vi "XML-compresion con etiquetas.vi"() -> ()   [LabVIEW 2010]
panel:
  out "temp 2":string="<?xml version=\"1.0\" encoding=\"UTF-8\"?><methodCall><methodName>jil.syncvi</methodName><params><param><value><array><value><struct><member><name>name</name><value><string>intin</string></value></member><member><name>action</name><value><string>set</string></value></member><member><name>value</name><value><int>0</int></value></member></struct></value><value><struct><member><name>name</name><value><string>doublein</string></value></member><member><name>action</name><value><string>set</string></value></member><member><name>value</name><value><double>0,000000</double></value></member></struct></value><value><struct><member><name>name</name><value><string>booleanin</string></value></member><member><name>action</name><value><string>set</string></value></member><member><name>value</name><value><boolean>1</boolean></value></member></struct></value><value><struct><member><name>name</name><value><string>stringin</string></value></member><member><name>action</name><value><string>set</string></value></member><member><name>value</name><value><string></string></value></member></struct></value><value><struct><member><name>name</name><value><string>intout</string></value></member><member><name>action</name><value><string>get</string></value></member><member><name>value</name><value><int>0</int></value></member></struct></value><value><struct><member><name>name</name><value><string>doubleout</string></value></member><member><name>action</name><value><string>get</string></value></member><member><name>value</name><value><double>0</double></value></member></struct></value><value><struct><member><name>name</name><value><string>booleanout</string></value></member><member><name>action</name><value><string>get</string></value></member><member><name>value</name><value><boolean>0</boolean></value></member></struct></value><value><struct><member><name>name</name><value><string>stringout</string></value></member><member><name>action</name><value><string>get</string></value></member><member><name>value</name><value><string>a</string></value></member></struct></value></array></value></param></params></methodCall>"
  out "temp":string="<1>intin<2>set<3><8>0</8><4>doublein<2>set<3><6>0,000000</6><4>booleanin<2>set<3><5>1</5><4>stringin<2>set<3><7></7><4>intout<2>get<3><8>0</8><4>doubleout<2>get<3><6>0</6><4>booleanout<2>get<3><5>0</5><4>stringout<2>get<3><7>a</7></1>"
  in  "comprimido":string[](array[string])=["<1>", "</1>", "<2>", "<3>", "<4>", "<5>", "</5>", "<6>", "</6>", "<7>", "</7>", "<8>", "</8>"]
  in  "Expandido":string[](array[string])=["<?xml version=\"1.0\" encoding=\"UTF-8\"?><methodCall><methodName>jil.syncvi</methodName><params><param><value><array><value><struct><member><name>name</name><value><string>", "</value></member></struct></value></array></value></param></params></methodCall>", "</string></value></member><member><name>action</name><value><string>", "</string></value></member><member><name>value</name><value>", "</value></member></struct></value><value><struct><member><name>name</name><value><string>", "<boolean>", "</boolean>", "<double>", "</double>", "<string>", "</string>", "<int>", "</int>"]
  out "antes 2":string="<?xml version=\"1.0\" encoding=\"UTF-8\"?>\n<methodCall>\n<methodName>jil.syncvi</methodName>\n<params>\n<param>\n<value>\n<array>\n<value>\n<struct>\n<member>\n<name>name</name>\n<value>\n<string>intin</string>\n</value>\n</member>\n<member>\n<name>action</name>\n<value>\n<string>set</string>\n</value>\n</member>\n<member>\n<name>value</name>\n<value>\n<int>0</int>\n</value>\n</member>\n</struct>\n</value>\n<value>\n<struct>\n<member>\n<name>name</name>\n<value>\n<string>doublein</string>\n</value>\n</member>\n<member>\n<name>action</name>\n<value>\n<string>set</string>\n</value>\n</member>\n<member>\n<name>value</name>\n<value>\n<double>0,000000</double>\n</value>\n</member>\n</struct>\n</value>\n<value>\n<struct>\n<member>\n<name>name</name>\n<value>\n<string>booleanin</string>\n</value>\n</member>\n<member>\n<name>action</name>\n<value>\n<string>set</string>\n</value>\n</member>\n<member>\n<name>value</name>\n<value>\n<boolean>1</boolean>\n</value>\n</member>\n</struct>\n</value>\n<value>\n<struct>\n<member>\n<name>name</name>\n<value>\n<string>stringin</string>\n</value>\n</member>\n<member>\n<name>action</name>\n<value>\n<string>set</string>\n</value>\n</member>\n<member>\n<name>value</name>\n<value>\n<string></string>\n</value>\n</member>\n</struct>\n</value>\n<value>\n<struct>\n<member>\n<name>name</name>\n<value>\n<string>intout</string>\n</value>\n</member>\n<member>\n<name>action</name>\n<value>\n<string>get</string>\n</value>\n</member>\n<member>\n<name>value</name>\n<value>\n<int>0</int>\n</value>\n</member>\n</struct>\n</value>\n<value>\n<struct>\n<member>\n<name>name</name>\n<value>\n<string>doubleout</string>\n</value>\n</member>\n<member>\n<name>action</name>\n<value>\n<string>get</string>\n</value>\n</member>\n<member>\n<name>value</name>\n<value>\n<double>0</double>\n</value>\n</member>\n</struct>\n</value>\n<value>\n<struct>\n<member>\n<name>name</name>\n<value>\n<string>booleanout</string>\n</value>\n</member>\n<member>\n<name>action</name>\n<value>\n<string>get</string>\n</value>\n</member>\n<member>\n<name>value</name>\n<value>\n<boolean>0</boolean>\n</value>\n</member>\n</struct>\n</value>\n<value>\n<struct>\n<member>\n<name>name</name>\n<value>\n<string>stringout</string>\n</value>\n</member>\n<member>\n<name>action</name>\n<value>\n<string>get</string>\n</value>\n</member>\n<member>\n<name>value</name>\n<value>\n<string>a</string>\n</value>\n</member>\n</struct>\n</value>\n</array>\n</value>\n</param>\n</params>\n</methodCall>"
  out "despues 2":string
  out "despues":string
  out "Mensaje LEGIBLE DESC":string="<?xml version=\"1.0\" encoding=\"UTF-8\"?>\n<methodCall>\n<methodName>jil.syncvi</methodName>\n<params>\n<param>\n<value>\n<array>\n<value>\n<struct>\n<member>\n<name>name</name>\n<value>\n<string>intin</string>\n</value>\n</member>\n<member>\n<name>action</name>\n<value>\n<string>set</string>\n</value>\n</member>\n<member>\n<name>value</name>\n<value>\n<int>0</int>\n</value>\n</member>\n</struct>\n</value>\n<value>\n<struct>\n<member>\n<name>name</name>\n<value>\n<string>doublein</string>\n</value>\n</member>\n<member>\n<name>action</name>\n<value>\n<string>set</string>\n</value>\n</member>\n<member>\n<name>value</name>\n<value>\n<double>0,000000</double>\n</value>\n</member>\n</struct>\n</value>\n<value>\n<struct>\n<member>\n<name>name</name>\n<value>\n<string>booleanin</string>\n</value>\n</member>\n<member>\n<name>action</name>\n<value>\n<string>set</string>\n</value>\n</member>\n<member>\n<name>value</name>\n<value>\n<boolean>1</boolean>\n</value>\n</member>\n</struct>\n</value>\n<value>\n<struct>\n<member>\n<name>name</name>\n<value>\n<string>stringin</string>\n</value>\n</member>\n<member>\n<name>action</name>\n<value>\n<string>set</string>\n</value>\n</member>\n<member>\n<name>value</name>\n<value>\n<string></string>\n</value>\n</member>\n</struct>\n</value>\n<value>\n<struct>\n<member>\n<name>name</name>\n<value>\n<string>intout</string>\n</value>\n</member>\n<member>\n<name>action</name>\n<value>\n<string>get</string>\n</value>\n</member>\n<member>\n<name>value</name>\n<value>\n<int>0</int>\n</value>\n</member>\n</struct>\n</value>\n<value>\n<struct>\n<member>\n<name>name</name>\n<value>\n<string>doubleout</string>\n</value>\n</member>\n<member>\n<name>action</name>\n<value>\n<string>get</string>\n</value>\n</member>\n<member>\n<name>value</name>\n<value>\n<double>0</double>\n</value>\n</member>\n</struct>\n</value>\n<value>\n<struct>\n<member>\n<name>name</name>\n<value>\n<string>booleanout</string>\n</value>\n</member>\n<member>\n<name>action</name>\n<value>\n<string>get</string>\n</value>\n</member>\n<member>\n<name>value</name>\n<value>\n<boolean>0</boolean>\n</value>\n</member>\n</struct>\n</value>\n<value>\n<struct>\n<member>\n<name>name</name>\n<value>\n<string>stringout</string>\n</value>\n</member>\n<member>\n<name>action</name>\n<value>\n<string>get</string>\n</value>\n</member>\n<member>\n<name>value</name>\n<value>\n<string>a</string>\n</value>\n</member>\n</struct>\n</value>\n</array>\n</value>\n</param>\n</params>\n</methodCall>"
  out "Tiempo que tarda\nen comprimir y descomorimir (ms)":dbl=1.068
  out "OK?":bool=TRUE
  out "MensajeDESC":string="<?xml version=\"1.0\" encoding=\"UTF-8\"?><methodCall><methodName>jil.syncvi</methodName><params><param><value><array><value><struct><member><name>name</name><value><string>intin</string></value></member><member><name>action</name><value><string>set</string></value></member><member><name>value</name><value><int>0</int></value></member></struct></value><value><struct><member><name>name</name><value><string>doublein</string></value></member><member><name>action</name><value><string>set</string></value></member><member><name>value</name><value><double>0,000000</double></value></member></struct></value><value><struct><member><name>name</name><value><string>booleanin</string></value></member><member><name>action</name><value><string>set</string></value></member><member><name>value</name><value><boolean>1</boolean></value></member></struct></value><value><struct><member><name>name</name><value><string>stringin</string></value></member><member><name>action</name><value><string>set</string></value></member><member><name>value</name><value><string></string></value></member></struct></value><value><struct><member><name>name</name><value><string>intout</string></value></member><member><name>action</name><value><string>get</string></value></member><member><name>value</name><value><int>0</int></value></member></struct></value><value><struct><member><name>name</name><value><string>doubleout</string></value></member><member><name>action</name><value><string>get</string></value></member><member><name>value</name><value><double>0</double></value></member></struct></value><value><struct><member><name>name</name><value><string>booleanout</string></value></member><member><name>action</name><value><string>get</string></value></member><member><name>value</name><value><boolean>0</boolean></value></member></struct></value><value><struct><member><name>name</name><value><string>stringout</string></value></member><member><name>action</name><value><string>get</string></value></member><member><name>value</name><value><string>a</string></value></member></struct></value></array></value></param></params></methodCall>"
  out "length 3":i32=234
  out "Mensaje3":string="<1>intin<2>set<3><8>0</8><4>doublein<2>set<3><6>0,000000</6><4>booleanin<2>set<3><5>1</5><4>stringin<2>set<3><7></7><4>intout<2>get<3><8>0</8><4>doubleout<2>get<3><6>0</6><4>booleanout<2>get<3><5>0</5><4>stringout<2>get<3><7>a</7></1>"
  out "length 2":i32=2118
  out "Mensaje2":string="<?xml version=\"1.0\" encoding=\"UTF-8\"?><methodCall><methodName>jil.syncvi</methodName><params><param><value><array><value><struct><member><name>name</name><value><string>intin</string></value></member><member><name>action</name><value><string>set</string></value></member><member><name>value</name><value><int>0</int></value></member></struct></value><value><struct><member><name>name</name><value><string>doublein</string></value></member><member><name>action</name><value><string>set</string></value></member><member><name>value</name><value><double>0,000000</double></value></member></struct></value><value><struct><member><name>name</name><value><string>booleanin</string></value></member><member><name>action</name><value><string>set</string></value></member><member><name>value</name><value><boolean>1</boolean></value></member></struct></value><value><struct><member><name>name</name><value><string>stringin</string></value></member><member><name>action</name><value><string>set</string></value></member><member><name>value</name><value><string></string></value></member></struct></value><value><struct><member><name>name</name><value><string>intout</string></value></member><member><name>action</name><value><string>get</string></value></member><member><name>value</name><value><int>0</int></value></member></struct></value><value><struct><member><name>name</name><value><string>doubleout</string></value></member><member><name>action</name><value><string>get</string></value></member><member><name>value</name><value><double>0</double></value></member></struct></value><value><struct><member><name>name</name><value><string>booleanout</string></value></member><member><name>action</name><value><string>get</string></value></member><member><name>value</name><value><boolean>0</boolean></value></member></struct></value><value><struct><member><name>name</name><value><string>stringout</string></value></member><member><name>action</name><value><string>get</string></value></member><member><name>value</name><value><string>a</string></value></member></struct></value></array></value></param></params></methodCall>"
  out "antes":string="<?xml version=\"1.0\" encoding=\"UTF-8\"?><methodCall><methodName>jil.syncvi</methodName><params><param><value><array><value><struct><member><name>name</name><value><string>intin</string></value></member><member><name>action</name><value><string>set</string></value></member><member><name>value</name><value><int>0</int></value></member></struct></value><value><struct><member><name>name</name><value><string>doublein</string></value></member><member><name>action</name><value><string>set</string></value></member><member><name>value</name><value><double>0,000000</double></value></member></struct></value><value><struct><member><name>name</name><value><string>booleanin</string></value></member><member><name>action</name><value><string>set</string></value></member><member><name>value</name><value><boolean>1</boolean></value></member></struct></value><value><struct><member><name>name</name><value><string>stringin</string></value></member><member><name>action</name><value><string>set</string></value></member><member><name>value</name><value><string></string></value></member></struct></value><value><struct><member><name>name</name><value><string>intout</string></value></member><member><name>action</name><value><string>get</string></value></member><member><name>value</name><value><int>0</int></value></member></struct></value><value><struct><member><name>name</name><value><string>doubleout</string></value></member><member><name>action</name><value><string>get</string></value></member><member><name>value</name><value><double>0</double></value></member></struct></value><value><struct><member><name>name</name><value><string>booleanout</string></value></member><member><name>action</name><value><string>get</string></value></member><member><name>value</name><value><boolean>0</boolean></value></member></struct></value><value><struct><member><name>name</name><value><string>stringout</string></value></member><member><name>action</name><value><string>get</string></value></member><member><name>value</name><value><string>a</string></value></member></struct></value></array></value></param></params></methodCall>"
  out "length":i32=3347
  in  "Mensaje":string="<?xml version=\"1.0\" encoding=\"UTF-8\"?>\n<methodCall>\n\t<methodName>jil.syncvi</methodName>\n<params>\n  <param>\n    <value>\n    <array>\n\n      <value>\n      <struct>\n        <member>\n          <name>name</name>\n          <value><string>intin</string></value>\n        </member>\n        <member>\n          <name>action</name>\n          <value><string>set</string></value>\n        </member>\n        <member>\n          <name>value</name>\n          <value><int>0</int></value>\n        </member>\n      </struct>\n      </value>\n\n\n      <value>\n      <struct>\n        <member>\n          <name>name</name>\n          <value><string>doublein</string></value>\n        </member>\n        <member>\n          <name>action</name>\n          <value><string>set</string></value>\n        </member>\n        <member>\n          <name>value</name>\n          <value><double>0,000000</double></value>\n        </member>\n      </struct>\n      </value>\n\n      <value>\n      <struct>\n        <member>\n          <name>name</name>\n          <value><string>booleanin</string></value>\n        </member>\n        <member>\n          <name>action</name>\n          <value><string>set</string></value>\n        </member>\n        <member>\n          <name>value</name>\n          <value><boolean>1</boolean></value>\n        </member>\n      </struct>\n      </value>\n\n      <value>\n      <struct>\n        <member>\n          <name>name</name>\n          <value><string>stringin</string></value>\n        </member>\n        <member>\n          <name>action</name>\n          <value><string>set</string></value>\n        </member>\n        <member>\n          <name>value</name>\n          <value><string></string></value>\n        </member>\n      </struct>\n      </value>\n\n\n      <value>\n      <struct>\n        <member>\n          <name>name</name>\n          <value><string>intout</string></value>\n        </member>\n        <member>\n          <name>action</name>\n          <value><string>get</string></value>\n        </member>\n        <member>\n          <name>value</name>\n          <value><int>0</int></value>\n        </member>\n      </struct>\n      </value>\n\n\n      <value>\n      <struct>\n        <member>\n          <name>name</name>\n          <value><string>doubleout</string></value>\n        </member>\n        <member>\n          <name>action</name>\n          <value><string>get</string></value>\n        </member>\n        <member>\n          <name>value</name>\n          <value><double>0</double></value>\n        </member>\n      </struct>\n      </value>\n\n      <value>\n      <struct>\n        <member>\n          <name>name</name>\n          <value><string>booleanout</string></value>\n        </member>\n        <member>\n          <name>action</name>\n          <value><string>get</string></value>\n        </member>\n        <member>\n          <name>value</name>\n          <value><boolean>0</boolean></value>\n        </member>\n      </struct>\n      </value>\n\n      <value>\n      <struct>\n        <member>\n          <name>name</name>\n          <value><string>stringout</string></value>\n        </member>\n        <member>\n          <name>action</name>\n          <value><string>get</string></value>\n        </member>\n        <member>\n          <name>value</name>\n          <value><string>a</string></value>\n        </member>\n      </struct>\n      </value>\n\n\n    </array>\n    </value>\n  </param>\n</params>\n</methodCall>"
  # "comprimiendo con rar llega  a 412"
  # "Este es un ejemplo sencillo de compresion por etiquetas"
  # "sin espacios"
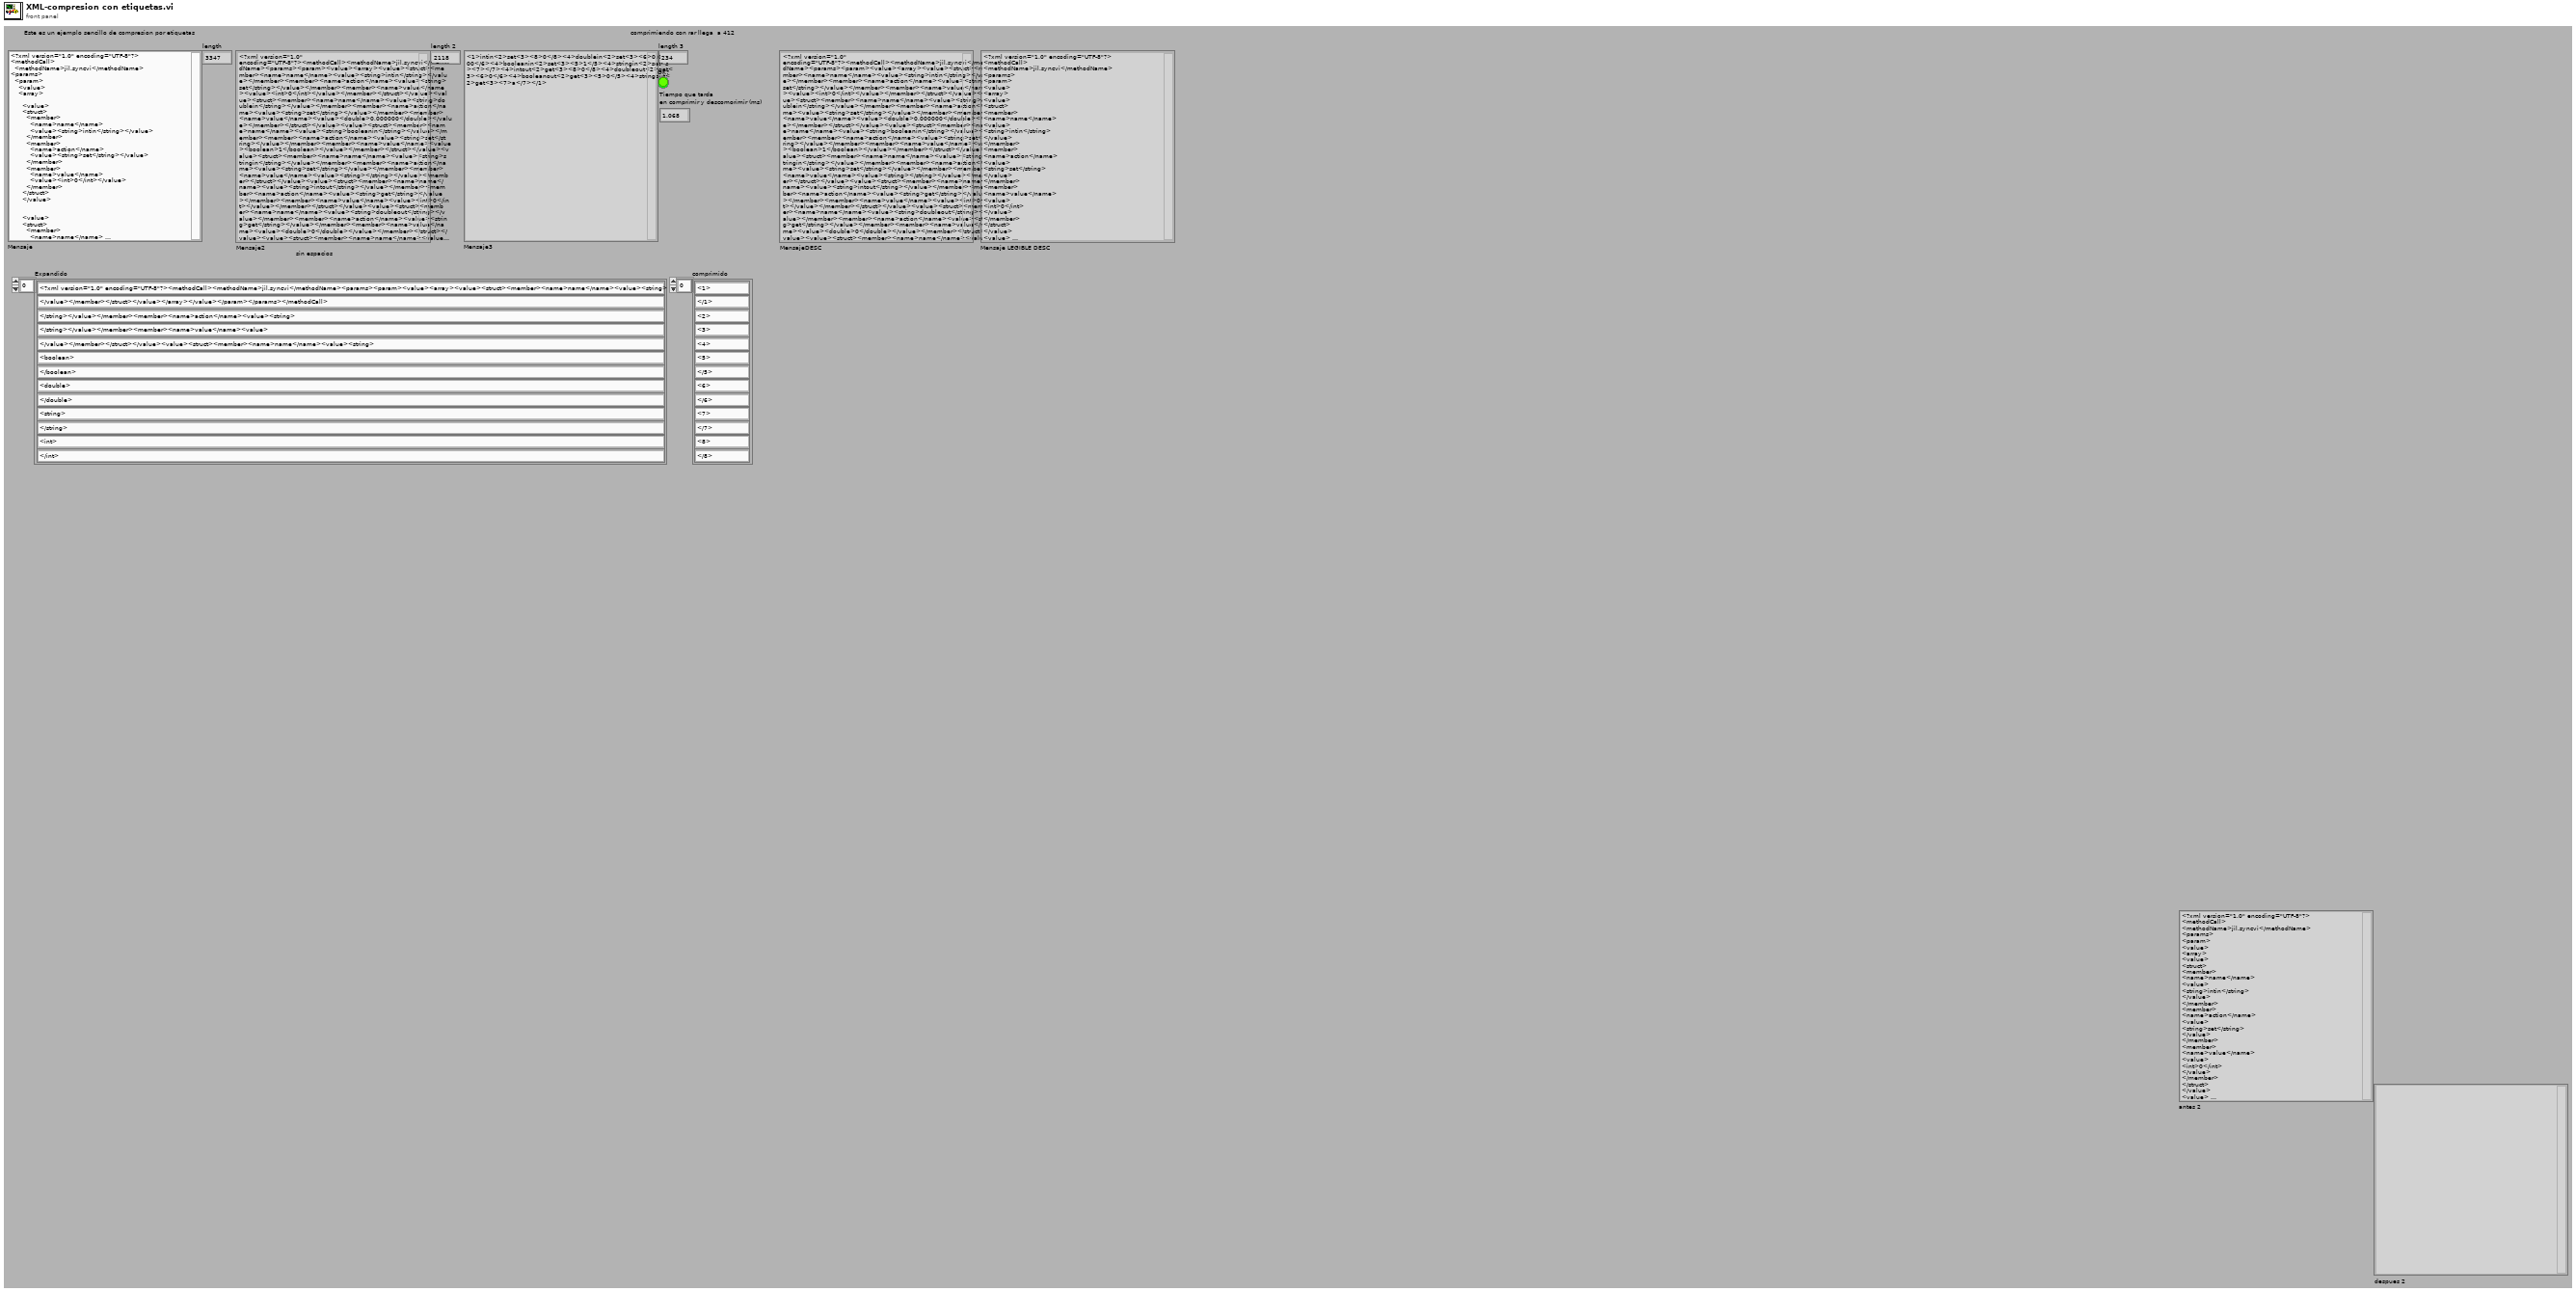
[diagram p1: front panel]
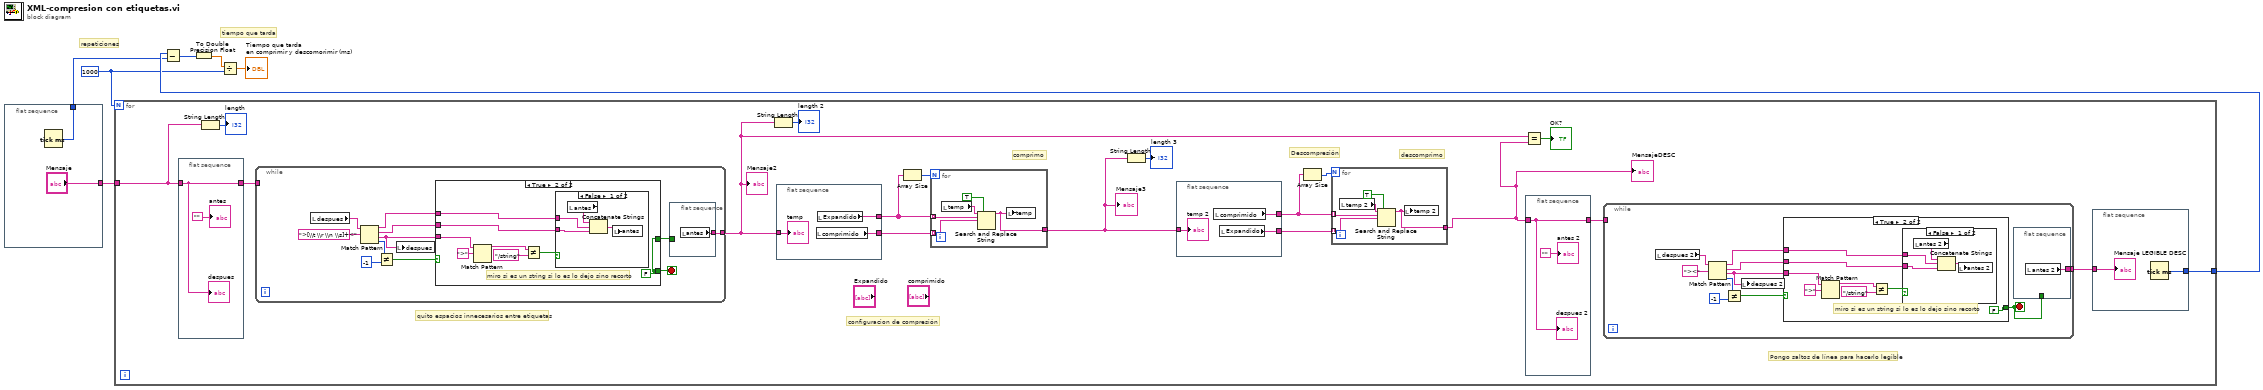
[diagram p0: block diagram]
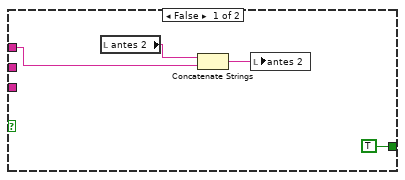
[diagram p2: hidden frame]
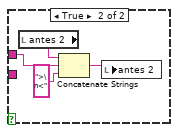
[diagram p3: hidden frame]
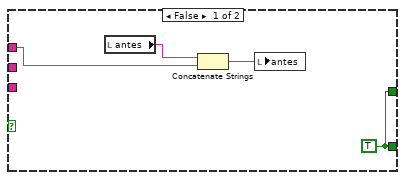
[diagram p4: hidden frame]
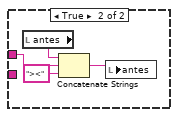
[diagram p5: hidden frame]
diagram:
  w2 = 1000
  # "repeticiones"
  # "tiempo que tarda"
  n1 = flat-sequence {
    tunnel: ["Mensaje"] -> w7
    tunnel: [w8] -> w5
    frame #0 {
      n2 = Tick Count (ms)() -> (millisecond timer value=w8:u32)
    }
  }
  n3 = for {
    N: w2 -> [_]
    tunnel: w7 -> [w26]
    tunnel: [w22] -> w6
    # "Pongo saltos de línea para hacerlo legible"
    # "descomprimo"
    # "comprimo"
    # "configuracion de compresión"
    # "quito espacios innecesarios entre etiquetas"
    # "Descompresión"
    n4 = flat-sequence {
      tunnel: [w112] -> w21
      tunnel: w26 -> [w112]
      frame #0 {
        "antes" <- ""
        "despues" <- w112
      }
    }
    n5 = String Length(string=w26) -> (length=→"length":i32)
    n6 = while {
      tunnel: w21 -> [_]
      tunnel: [w80] -> w18
      stop <- w81 stop-if-true
      n7 = local read "despues"() -> (w87:string)
      n8 = Match Pattern(string=w87, regular expression=">[\\t \\r \\n \\s]+<") -> (before substring=w84:string, match substring=w83:string, after substring=w82:string, offset past match=w89:i32)  [unwired: 1 in]
      n9 = Not Equal?(x=w89, y=-1) -> (x != y?=w85:bool)
      n10 = local write "despues"(w82) -> ()
      n11 = case shown="True" w85 {
        tunnel: w84 -> [w92 w97]
        tunnel: w83 -> [_ w96]
        tunnel: w82 -> [_ w99]
        tunnel: [w91 w95] -> w81
        tunnel: [w91 w95] -> w79
        frame False {
          w91 = TRUE
          n12 = local read "antes"() -> (w93:string)
          n13 = Concatenate Strings(w93, w92) -> (w94:string)
          n14 = local write "antes"(w94) -> ()
        }
        frame True {
          w95 = FALSE
          # "miro si es un string si lo es lo dejo sino recorto"
          n15 = Match Pattern(string=w99, regular expression=">") -> (before substring=w101:string)  [unwired: 1 in, 3 out]
          n16 = Not Equal?(x=w101, y="/string") -> (x != y?=w98:bool)
          n17 = case shown="False" w98 {
            tunnel: w97 -> [w106 w110]
            tunnel: w96 -> [w105 _]
            frame False {
              n18 = local read "antes"() -> (w103:string)
              n19 = Concatenate Strings(w103, w106, w105) -> (w104:string)
              n20 = local write "antes"(w104) -> ()
            }
            frame True {
              n21 = local read "antes"() -> (w107:string)
              n22 = Concatenate Strings(w107, w110, "><" ("string")) -> (w108:string)
              n23 = local write "antes"(w108) -> ()
            }
          }
        }
      }
      n24 = flat-sequence {
        tunnel: [w90] -> w80
        tunnel: w79 -> [_]
        frame #0 {
          n25 = local read "antes"() -> (w90:string)
        }
      }
    }
    "Mensaje2" <- w18
    n26 = String Length(string=w18) -> (length=→"length 2":i32)
    n27 = flat-sequence {
      tunnel: w18 -> [w40]
      tunnel: [w39] -> w16
      tunnel: [w38] -> w15
      frame #0 {
        n28 = local read "comprimido"() -> (w39:string[])
        n29 = local read "Expandido"() -> (w38:string[])
        "temp" <- w40
      }
    }
    n30 = Array Size(array=w15) -> (size(s)=w17:i32)
    n31 = for {
      N: w17 -> [_]
      tunnel: w15 -> [w44] mode=indexing
      tunnel: w16 -> [w43] mode=indexing
      tunnel: [w42] -> w11
      n32 = local read "temp"() -> (w45:string)
      n33 = Search and Replace String(replace all?=TRUE ("replace all? (F)"), input string=w45, search string=w44, replace string=w43) -> (result string=w42:string)  [unwired: 4 in, 3 out]
      n34 = local write "temp"(w42) -> ()
    }
    "Mensaje3" <- w11
    n35 = String Length(string=w11) -> (length=→"length 3":i32)
    n36 = flat-sequence {
      tunnel: w11 -> [w32]
      tunnel: [w31] -> w13
      tunnel: [w30] -> w12
      frame #0 {
        n37 = local read "comprimido"() -> (w30:string[])
        n38 = local read "Expandido"() -> (w31:string[])
        "temp 2" <- w32
      }
    }
    n39 = Array Size(array=w12) -> (size(s)=w14:i32)
    n40 = for {
      N: w14 -> [_]
      tunnel: w12 -> [w36] mode=indexing
      tunnel: w13 -> [w35] mode=indexing
      tunnel: [w34] -> w10
      n41 = local read "temp 2"() -> (w37:string)
      n42 = Search and Replace String(replace all?=TRUE ("replace all? (F)"), input string=w37, search string=w36, replace string=w35) -> (result string=w34:string)  [unwired: 4 in, 3 out]
      n43 = local write "temp 2"(w34) -> ()
    }
    "MensajeDESC" <- w10
    n44 = Equal?(x=w18, y=w10) -> (x = y?=→"OK?":bool)
    n45 = flat-sequence {
      tunnel: [w78] -> w20
      tunnel: w10 -> [w78]
      frame #0 {
        "antes 2" <- ""
        "despues 2" <- w78
      }
    }
    n46 = while {
      tunnel: w20 -> [_]
      tunnel: [w47] -> w19
      stop <- w46 stop-if-true
      n47 = local read "despues 2"() -> (w53:string)
      n48 = Match Pattern(string=w53, regular expression="><") -> (before substring=w50:string, match substring=w49:string, after substring=w48:string, offset past match=w55:i32)  [unwired: 1 in]
      n49 = Not Equal?(x=w55, y=-1) -> (x != y?=w51:bool)
      n50 = local write "despues 2"(w48) -> ()
      n51 = case shown="True" w51 {
        tunnel: w50 -> [w57 w63]
        tunnel: w49 -> [_ w62]
        tunnel: w48 -> [_ w65]
        tunnel: [TRUE FALSE] -> w46
        frame False {
          n52 = local read "antes 2"() -> (w58:string)
          n53 = Concatenate Strings(w58, w57) -> (w59:string)
          n54 = local write "antes 2"(w59) -> ()
        }
        frame True {
          # "miro si es un string si lo es lo dejo sino recorto"
          n55 = Match Pattern(string=w65, regular expression=">") -> (before substring=w67:string)  [unwired: 1 in, 3 out]
          n56 = Not Equal?(x=w67, y="/string") -> (x != y?=w64:bool)
          n57 = case shown="False" w64 {
            tunnel: w63 -> [w72 w76]
            tunnel: w62 -> [w71 _]
            frame False {
              n58 = local read "antes 2"() -> (w69:string)
              n59 = Concatenate Strings(w69, w72, w71) -> (w70:string)
              n60 = local write "antes 2"(w70) -> ()
            }
            frame True {
              n61 = local read "antes 2"() -> (w73:string)
              n62 = Concatenate Strings(w73, w76, ">\n<" ("string")) -> (w74:string)
              n63 = local write "antes 2"(w74) -> ()
            }
          }
        }
      }
      n64 = flat-sequence {
        tunnel: [w56] -> w47
        tunnel: w46 -> [_]
        frame #0 {
          n65 = local read "antes 2"() -> (w56:string)
        }
      }
    }
    n66 = flat-sequence {
      tunnel: [w29] -> w22
      tunnel: w19 -> [w28]
      frame #0 {
        n67 = Tick Count (ms)() -> (millisecond timer value=w29:u32)
        "Mensaje LEGIBLE DESC" <- w28
      }
    }
  }
  n68 = Subtract(x=w6, y=w5) -> (x-y=w4:u32)
  n69 = To Double Precision Float(number=w4) -> (double precision float=w3:dbl)
  n70 = Divide(x=w3, y=w2) -> (x/y=→"Tiempo que tarda\nen comprimir y descomorimir (ms)":dbl)
